vi "TensileFGV.vi"(7 "FGV_mods":T1, 8 "Error In":errorcluster, 11 "DataIn":variant) -> (0 "Error Out":errorcluster, 3 "DataOut":variant)   [LabVIEW 2016]
uses:
  FGV_mods.ctl
  FGV_data.ctl
  TypeDefs/specimen_data.ctl
  TypeDefs/specimen_info.ctl
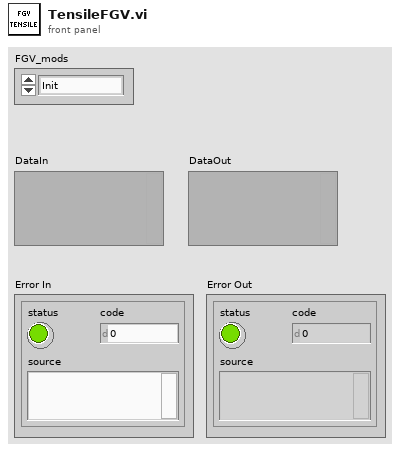
[diagram p1: front panel]
types:
  T1 = typedef "FGV_mods.ctl" = enum16{"Init", "read_headers", "read_file", "plot", "process", "End"}
  T2 = typedef "FGV_data.ctl" = cluster{"test_file":path, "specimens":T3[], "mean_strain":dbl[], "mean_stress":dbl[], "specimen_info":T4[]}
  T3 = typedef "specimen_data.ctl" = cluster{"time":dbl[], "extension":dbl[], "strain":dbl[], "load":dbl[], "stress":dbl[]}
  T4 = typedef "specimen_info.ctl" = cluster{"E":dbl, "Sy":dbl, "Sut":dbl, "eps max":dbl}
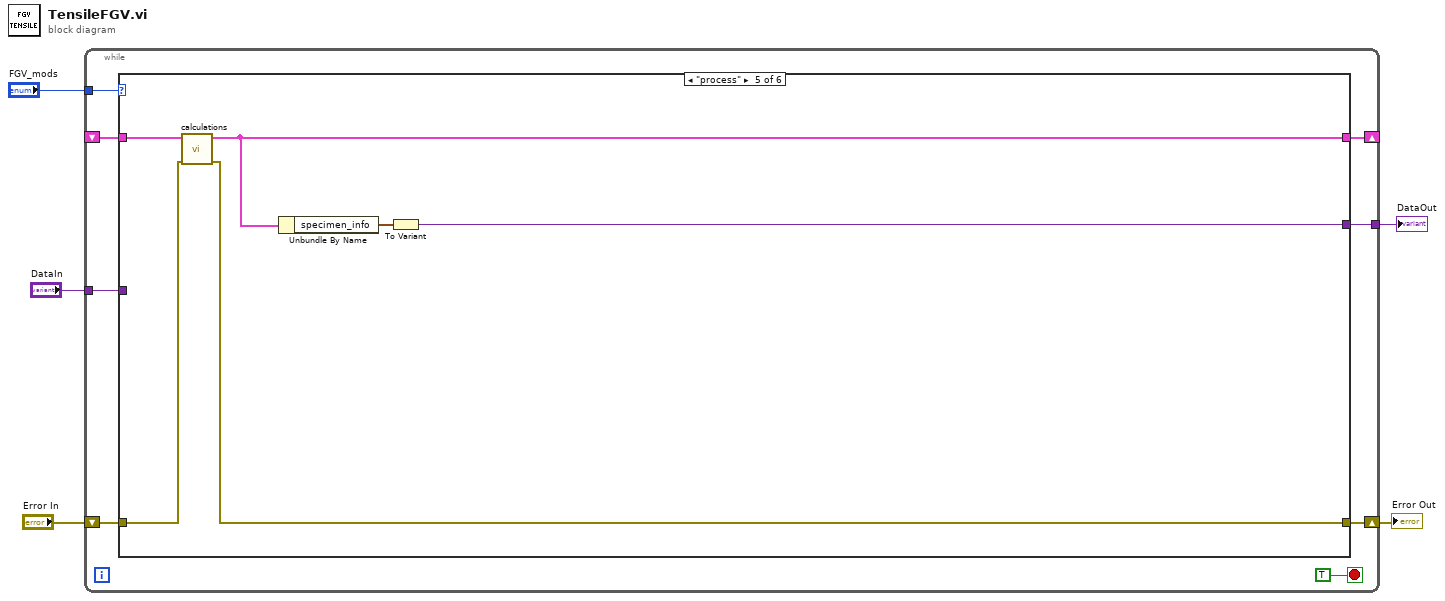
[diagram p0: block diagram]
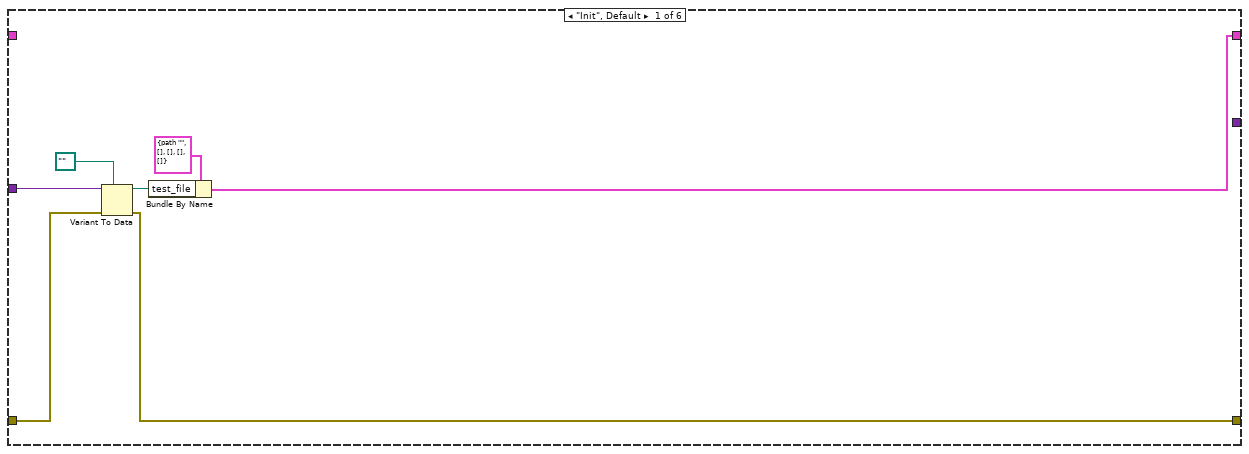
[diagram p2: hidden frame]
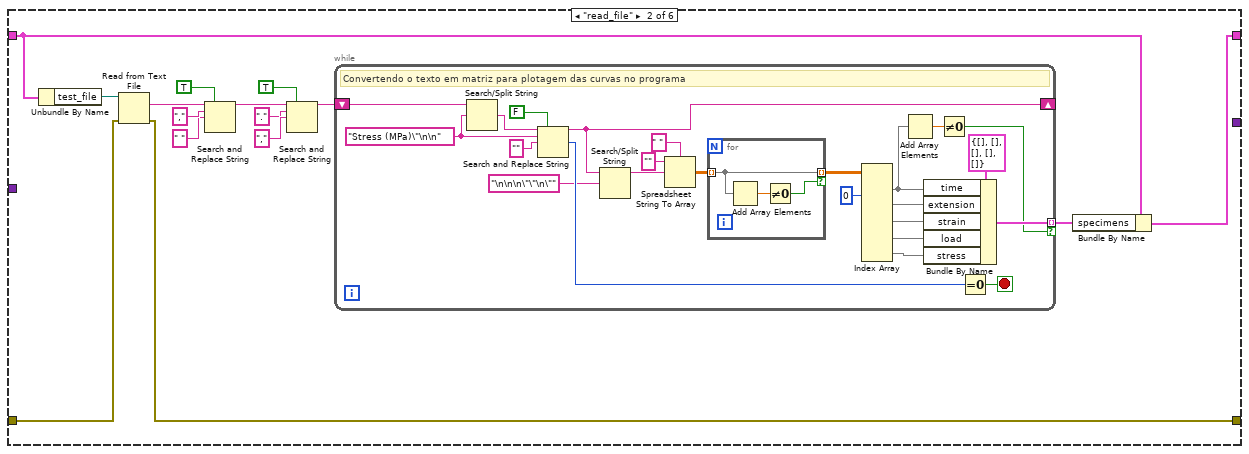
[diagram p3: hidden frame]
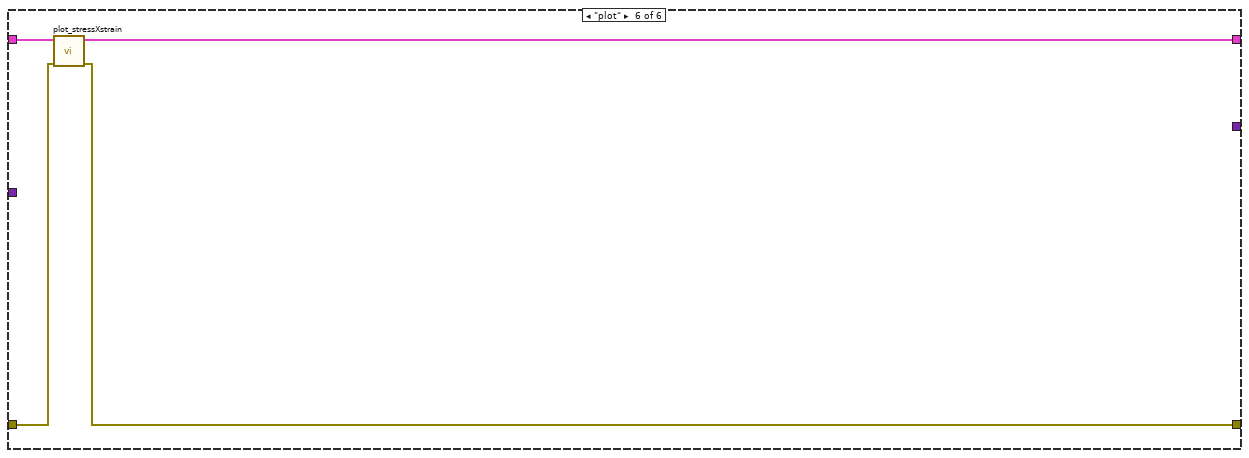
[diagram p6: hidden frame]
diagram:
  n1 = while {
    tunnel: "DataIn" -> [w12]
    tunnel: "FGV_mods" -> [w11]
    shift-right: [w10] -> _
    shift-left: _ -> [w9]
    shift-right: [w7] -> w2
    shift-left: "Error In" -> [w8]
    tunnel: [w6] -> w1
    stop <- TRUE stop-if-true
    n2 = case shown="\"process\"" w11 {
      tunnel: w12 -> [w20 _ _ _ _ _]
      tunnel: [w15 w21 w64 w66 w69 w73] -> w10
      tunnel: w9 -> [_ w23 w64 w66 w72 w76]
      tunnel: w8 -> [w19 w25 w63 w65 w71 w75]
      tunnel: [w14 w24 w63 w65 w70 w74] -> w7
      tunnel: [_ _ _ _ w67 _] -> w6
      frame "Init", Default {
        n3 = Variant To Data(error in=w19, type=path "", Variant=w20) -> (data=w17:path, error out=w14:errorcluster)
        n4 = Bundle By Name(cluster=T2 {"test_file"=path "", "specimens"=[], "mean_strain"=[], "mean_stress"=[], "specimen_info"=[]} ("FGV_data"), "test_file"=w17) -> (w15:T2)
      }
      frame "read_file" {
        n5 = Unbundle By Name(w23) -> ("test_file"=w26:path)
        n6 = Read from Text File(file (use dialog)=w26, error in=w25) -> (text=w35:string, error out=w24:errorcluster)  [unwired: 2 in, 2 out]
        n7 = Search and Replace String(replace all?=TRUE ("replace all? (F)"), input string=w35, search string=",", replace string=" " ("replace string (\"\")")) -> (result string=w30:string)  [unwired: 4 in, 3 out]
        n8 = Search and Replace String(replace all?=TRUE ("replace all? (F)"), input string=w30, search string=".", replace string="," ("replace string (\"\")")) -> (result string=w27:string)  [unwired: 4 in, 3 out]
        n9 = while {
          shift-right: [w48] -> _
          shift-left: w27 -> [w59]
          tunnel: [w43] -> w22 mode=indexing if=w38
          stop <- w53 stop-if-true
          w55 = "Stress (MPa)\"\n\n" ("search string/char (-)")
          # "Convertendo o texto em matriz para plotagem das curvas no programa"
          n10 = Search/Split String(string=w59, search string/char (-)=w55) -> (match + rest of string=w58:string)  [unwired: 1 in, 2 out]
          n11 = Search and Replace String(replace all?=FALSE ("replace all? (F)"), input string=w58, search string=w55, replace string="" ("replace string (\"\")")) -> (result string=w48:string, number of replacements=w54:i32)  [unwired: 4 in, 2 out]
          n12 = Search/Split String(string=w48, search string/char (-)="\n\n\n\"\"\n\"") -> (substring before match=w49:string)  [unwired: 1 in, 2 out]
          n13 = Spreadsheet String To Array(delimiter (Tab)=" ", format string="", spreadsheet string=w49) -> (array=w37:dbl[][])  [unwired: 1 in]
          n14 = for {
            tunnel: w37 -> [w61] mode=indexing
            tunnel: [w61] -> w36 mode=indexing if=w60
            n15 = Add Array Elements(numeric array=w61) -> (sum=w62:dbl)
            n16 = Not Equal To 0?(x=w62) -> (x != 0?=w60:bool)
          }
          n17 = Index Array(array=w36, index (col) #1=0 ("disabled index (col)")) -> (element #1=w40:dbl[], element #2=w46:dbl[], element #3=w45:dbl[], element #4=w44:dbl[], element #5=w41:dbl[])  [unwired: 9 in]
          n18 = Add Array Elements(numeric array=w40) -> (sum=w39:dbl)
          n19 = Bundle By Name(cluster=T3 {"time"=[], "extension"=[], "strain"=[], "load"=[], "stress"=[]} ("specimen_data"), "time"=w40, "extension"=w46, "strain"=w45, "load"=w44, "stress"=w41) -> (w43:T3)
          n20 = Not Equal To 0?(x=w39) -> (x != 0?=w38:bool)
          n21 = Equal To 0?(x=w54) -> (x = 0?=w53:bool)
        }
        n22 = Bundle By Name(cluster=w23, "specimens"=w22) -> (w21:T2)
      }
      frame "End" {
      }
      frame "read_headers" {
      }
      frame "process" {
        n23 = call "calculations.vi"("error in"=w71, "FGV_data"=w72) -> ("error out"=w70:errorcluster, "FGV_data_out"=w69:T2)  [unwired: 8 in]
        n24 = Unbundle By Name(w69) -> ("specimen_info"=w68:T4[])
        n25 = To Variant(anything=w68) -> (Variant=w67:variant)
      }
      frame "plot" {
        n26 = call "plot_stressXstrain.vi"("error in"=w75, "FGV_data"=w76) -> ("error out"=w74:errorcluster, "FGV_data_out"=w73:T2)  [unwired: 8 in]
      }
    }
  }
  "DataOut" <- w1
  "Error Out" <- w2
